vi "WriteSizeMat_1DArray_4DPoint-I32.vi"(6 "Channel":i32=1, 8 "error in":errorcluster, 9 "Height":i32, 10 "Width":i32, 11 "Array in":T1[](array[typedef])) -> (0 "error out":errorcluster, 3 "Array out":T1[](array[typedef]))   [LabVIEW 2020, in "OpenLvVision_OpenCv.lvlib"]
doc: "Write size of the datatype\nNo malleable to breake vi inlining!"
uses:
  OpenLvVision_OpenCv.lvlib
  TypeDef/Point/4D_PointI32.ctl
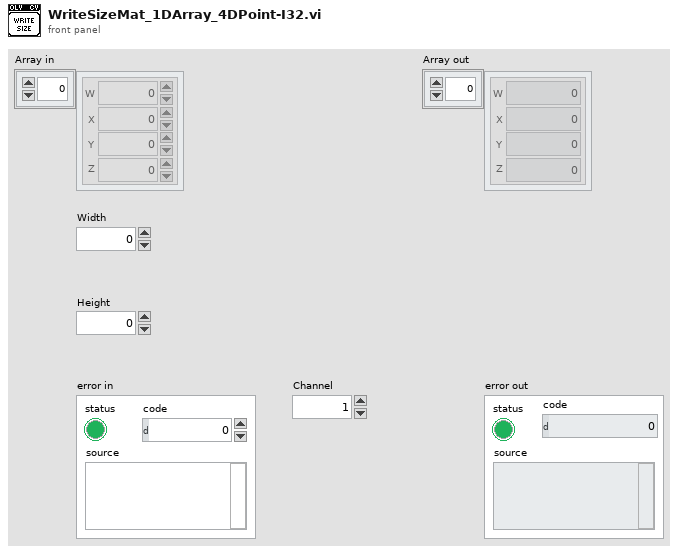
[diagram p1: front panel]
types:
  T1 = typedef "OpenLvVision_OpenCv.lvlib/4D_PointI32.ctl" = cluster{"W":i32, "X":i32, "Y":i32, "Z":i32}
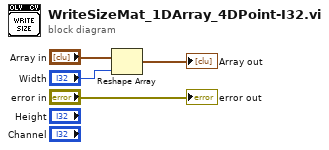
[diagram p0: block diagram]
diagram:
  n1 = Reshape Array("Array in", "Width") -> (→"Array out":T1[])
  "error out" <- "error in"
